vi "RT update 9219 parameters.vi"(3 "error in":errorcluster, 4 "FPGA Parameter cluster":T1={"Output settings"={"Relay Switch Matrix"=0, "Set output"=[0.0, 0.0, 0.0, 0.0], "set output?"=FALSE, "set relay matrix?"=FALSE}, "PID settings"={"PID input channel"=enum."PID Disabled", "PID output channel"=enum."PID Disabled", "PID gains"={"proportional gain"=0.0, "integral gain"=0.0, "derivative gain"=0.0, "filter coefficient"=0.0}, "PID output ranges"={"output high (Inf)"=0.0, "output low (-Inf)"=0.0}, "Setpoint for PID input chn"=0.0, "config PID gain?"=FALSE, "reset PID?"=FALSE, "config PID range?"=FALSE, "config PID input?"=FALSE, "config PID output?"=FALSE, "config PID setpoint?"=FALSE}, "NI9219 Settings"={"9219 Conversion Time"=enum."High Speed", "Input voltage range"=[0, 0, 0, 0], "config 9219 conversion time?"=FALSE, "config 9219 input range?"=FALSE}, "REQUEST_ID"=0, "requests"={"request_data"=FALSE, "request_system_status"=FALSE, "request_error_log"=FALSE}} {"REQUEST_ID" format="%x"; "NI9219 Settings"."Input voltage range" items=["+/- 60V", "+/- 15V", "+/- 4V", "+/- 1V", "+/- 125mV"]}, 5 "FPGA VI ref in":refnum<k20>) -> (0 "error out":errorcluster, 1 "FPGA Parameter cluster out":T1={"Output settings"={"Relay Switch Matrix"=0, "Set output"=[0.0, 0.0, 0.0, 0.0], "set output?"=FALSE, "set relay matrix?"=FALSE}, "PID settings"={"PID input channel"=enum."PID Disabled", "PID output channel"=enum."PID Disabled", "PID gains"={"proportional gain"=0.0, "integral gain"=0.0, "derivative gain"=0.0, "filter coefficient"=0.0}, "PID output ranges"={"output high (Inf)"=0.0, "output low (-Inf)"=0.0}, "Setpoint for PID input chn"=0.0, "config PID gain?"=FALSE, "reset PID?"=FALSE, "config PID range?"=FALSE, "config PID input?"=FALSE, "config PID output?"=FALSE, "config PID setpoint?"=FALSE}, "NI9219 Settings"={"9219 Conversion Time"=enum."High Speed", "Input voltage range"=[0, 0, 0, 0], "config 9219 conversion time?"=FALSE, "config 9219 input range?"=FALSE}, "REQUEST_ID"=0, "requests"={"request_data"=FALSE, "request_system_status"=FALSE, "request_error_log"=FALSE}} {"REQUEST_ID" format="%x"; "NI9219 Settings"."Input voltage range" items=["+/- 60V", "+/- 15V", "+/- 4V", "+/- 1V", "+/- 125mV"]}, 2 "FPGA VI Reference Out":refnum<k20>)   [LabVIEW 2018]
uses:
  Type Def Ctrls/RT ctrls/FPGA parameter cluster.ctl
  Type Def Ctrls/FPGA ctrls/NI9219VoltageRange.ctl
  <vilib>/Utility/error.llb/Error Cluster From Error Code.vi
  <vilib>/rvi/errors/niLvFpgaAdjustHostInterfaceError.vi
  <vilib>/rvi/interface/nirviReadWriteControl/nirviReadWriteControl.xnode
  NiFpgaLv.dll
  <vilib>/rvi/interface/Simulation/niFpgaSimulationCallBeginRW.vi
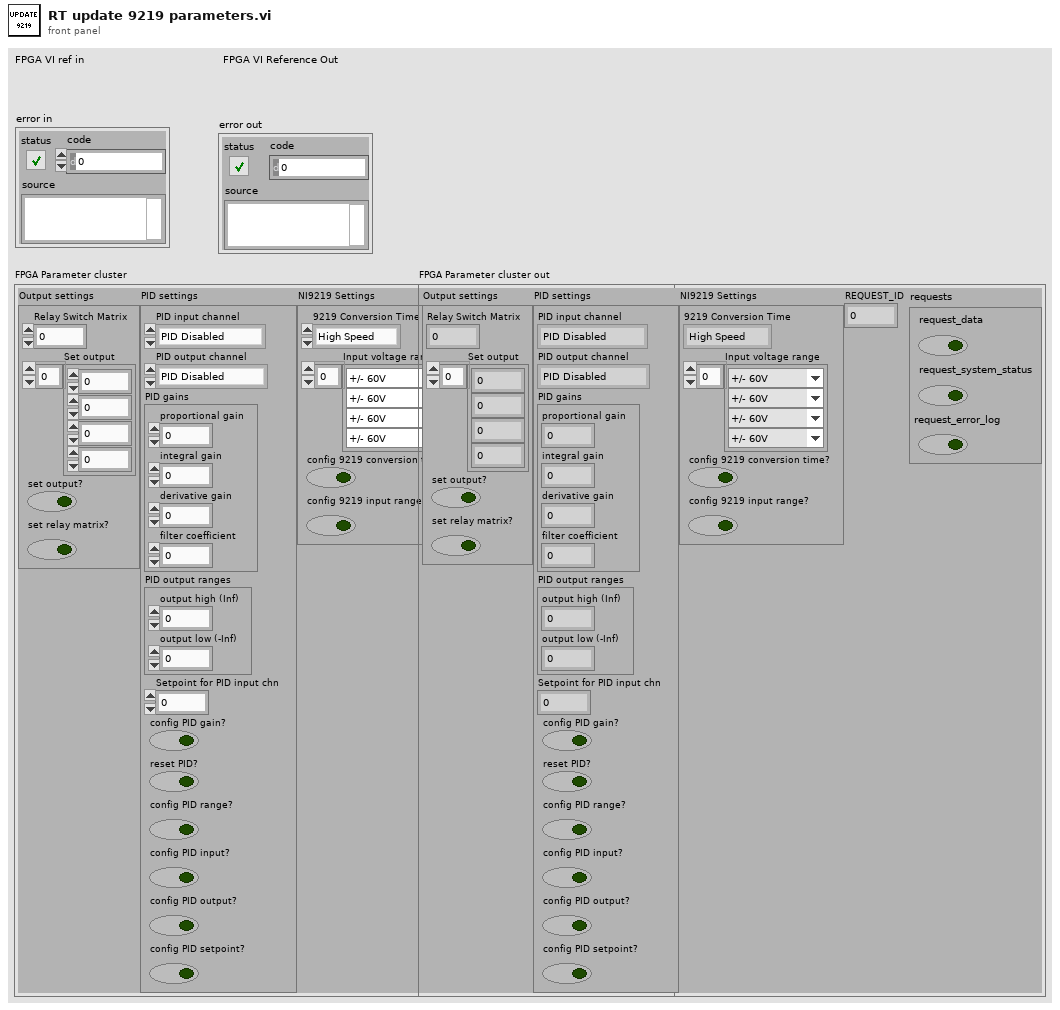
[diagram p1: front panel]
types:
  T1 = typedef "FPGA parameter cluster.ctl" = cluster{"Output settings":cluster{"Relay Switch Matrix":u32, "Set output":sgl[], "set output?":bool, "set relay matrix?":bool}, "PID settings":cluster{"PID input channel":enum16{"Output Channel 0", "Output Channel 1", "Output Channel 2", "Output Channel 3", "PID Disabled"}, "PID output channel":enum16{"Output Channel 0", "Output Channel 1", "Output Channel 2", "Output Channel 3", "PID Disabled"}, "PID gains":cluster{"proportional gain":sgl, "integral gain":sgl, "derivative gain":sgl, "filter coefficient":sgl}, "PID output ranges":cluster{"output high (Inf)":sgl, "output low (-Inf)":sgl}, "Setpoint for PID input chn":sgl, "config PID gain?":bool, "reset PID?":bool, "config PID range?":bool, "config PID input?":bool, "config PID output?":bool, "config PID setpoint?":bool}, "NI9219 Settings":cluster{"9219 Conversion Time":enum8{"High Speed", "Best 60 Hz Rejection", "Best 50 Hz Rejection", "High Resolution"}, "Input voltage range":T2[], "config 9219 conversion time?":bool, "config 9219 input range?":bool}, "REQUEST_ID":u64, "requests":cluster{"request_data":bool, "request_system_status":bool, "request_error_log":bool}}
  T2 = typedef "NI9219VoltageRange.ctl" = u8
  T3 = enum8{"High Speed", "Best 60 Hz Rejection", "Best 50 Hz Rejection", "High Resolution"}
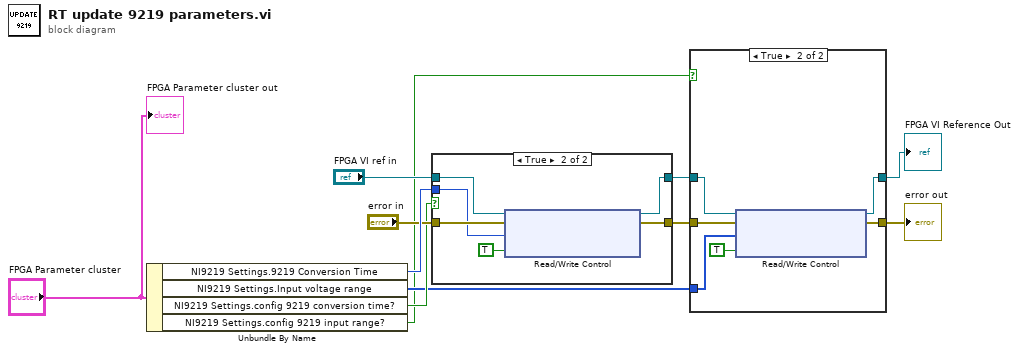
[diagram p0: block diagram]
diagram:
  n1 = Unbundle By Name("FPGA Parameter cluster") -> ("NI9219 Settings.9219 Conversion Time"=w11:T3, "NI9219 Settings.Input voltage range"=w6:T2[], "NI9219 Settings.config 9219 conversion time?"=w7:bool, "NI9219 Settings.config 9219 input range?"=w1:bool)
  n2 = case shown="True" w7 {
    tunnel: "FPGA VI ref in" -> [w13 w19]
    tunnel: [w13 w18] -> w5
    tunnel: "error in" -> [w12 w17]
    tunnel: [w12 w16] -> w4
    tunnel: w11 -> [_ w14]
    frame False {
    }
    frame True {
      n3 = xnode "Read/Write Control"("FPGA VI Reference In"=w19, "error in"=w17, "9219 Conversion Time"=w14, "Update  9219 settings"=TRUE) -> ("FPGA VI Reference Out"=w18:refnum<k20>, "error out"=w16:errorcluster)
    }
  }
  n4 = case shown="True" w1 {
    tunnel: [w21 w27] -> w3
    tunnel: [w20 w26] -> w2
    tunnel: w6 -> [_ w24]
    tunnel: w5 -> [w21 w23]
    tunnel: w4 -> [w20 w22]
    frame False {
    }
    frame True {
      n5 = xnode "Read/Write Control"("FPGA VI Reference In"=w23, "error in"=w22, "Input voltage range"=w24, "Update  9219 settings"=TRUE) -> ("FPGA VI Reference Out"=w27:refnum<k20>, "error out"=w26:errorcluster)
    }
  }
  "FPGA VI Reference Out" <- w3
  "error out" <- w2
  "FPGA Parameter cluster out" <- "FPGA Parameter cluster"
